vi "SendToSMGR.vi"(6 "error in":errorcluster, 7 "meas_point":i32, 8 "Files":path[](array[path]), 9 "max_value_":string[](array[string]) caption="max_values", 10 "microseconds":string="123456.7" caption="usec", 11 "date":string) -> (0 "error out":errorcluster, 2 "body":string, 3 "headers":string, 5 "time_shift":string="6")   [LabVIEW 2010]
uses:
  <vilib>/httpClient/MultipartData.ctl
  lib/Global 2.vi
  <vilib>/httpClient/LabVIEWHTTPClient.lvlib
panel:
  in  "Tab Control":enum32{"Page 1", "Page 2"}(tab)
  out "Array":T1[](array[typedef]) caption="Данные для формы"
  # "Запрос на добавление данных в базу на сервере\n---------------------------------------------------------------\nЕсли в ответе, в хедерсе есть строка \"HTTP/1.1 200 OK\"\nзначит всё действительно сделано правильно"
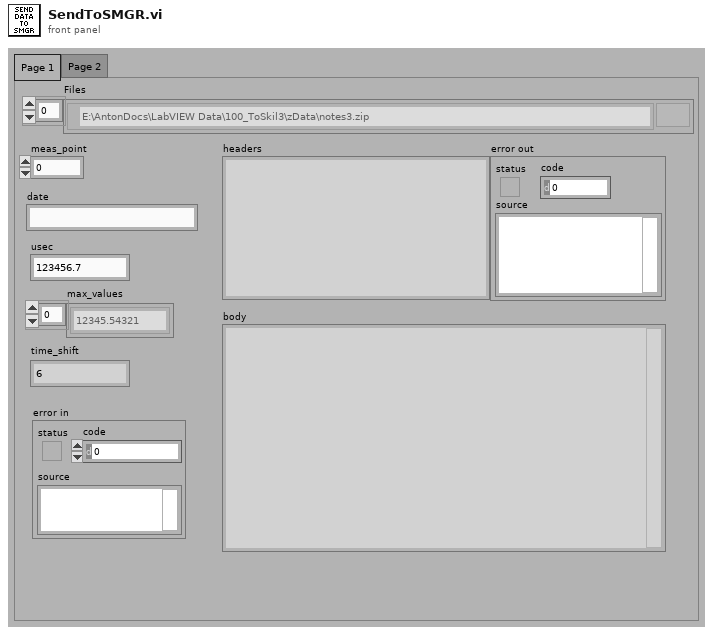
[diagram p1: front panel]
types:
  T1 = typedef "LabVIEWHTTPClient.lvlib/MultipartData.ctl" = cluster{"Name":string, "Value":string, "File":path, "Filename":string, "MIME type":string}
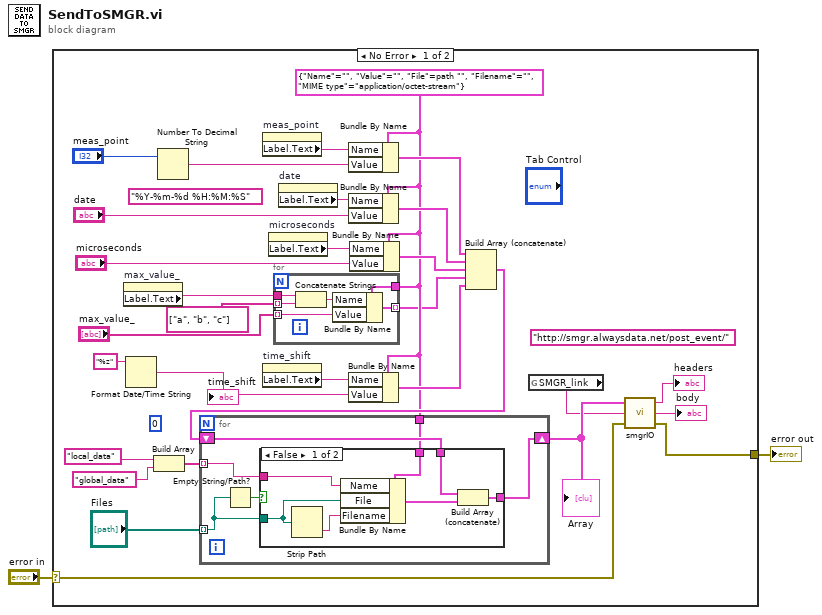
[diagram p0: block diagram]
diagram:
  n1 = case shown="No Error" "error in" {
    selector: "error in" -> [w6 w53]
    tunnel: [w3 w53] -> w1
    frame No Error {
      (unwired) 0
      w12 = T1 {"Name"="", "Value"="", "File"=path "", "Filename"="", "MIME type"="application/octet-stream"} ("postData")
      (unwired) "%Y-%m-%d %H:%M:%S" ("time format string (%c)")
      (unwired) "http://smgr.alwaysdata.net/post_event/" ("URL")
      n2 = property on="max_value_" class="Arr (strict)"() -> ("Label.Text"=w10:string)  [unwired: 2 in, 2 out]
      n3 = Format Date/Time String(time format string (%c)="%z") -> (date/time string=w14:string)  [unwired: 2 in]
      "time_shift" <- w14
      n4 = Build Array("local_data" ("Name"), "global_data" ("Name")) -> (w21:string[])
      n5 = Number To Decimal String(number="meas_point") -> (decimal integer string=w28:string)  [unwired: 1 in]
      n6 = property on="meas_point" class="DigNum (strict)"() -> ("Label.Text"=w19:string)  [unwired: 2 in, 2 out]
      n7 = property on="time_shift" class="Str"() -> ("Label.Text"=w20:string)  [unwired: 2 in, 2 out]
      n8 = property on="microseconds" class="Str"() -> ("Label.Text"=w17:string)  [unwired: 2 in, 2 out]
      n9 = for {
        tunnel: "max_value_" -> [w36] mode=indexing
        tunnel: w12 -> [w38]
        tunnel: [w37] -> w11 mode=indexing
        tunnel: w10 -> [w35]
        tunnel: string[] ["a", "b", "c"] -> [w34] mode=indexing
        n10 = Concatenate Strings(w35, w34) -> (w33:string)
        n11 = Bundle By Name(cluster=w38, "Name"=w33, "Value"=w36) -> (w37:T1)
      }
      n12 = property on="date" class="Str"() -> ("Label.Text"=w18:string)  [unwired: 2 in, 2 out]
      n13 = Bundle By Name(cluster=w12, "Name"=w19, "Value"=w28) -> (w32:T1)
      n14 = Bundle By Name(cluster=w12, "Name"=w18, "Value"="date") -> (w31:T1)
      n15 = Bundle By Name(cluster=w12, "Name"=w20, "Value"=w14) -> (w25:T1)
      n16 = Bundle By Name(cluster=w12, "Name"=w17, "Value"="microseconds") -> (w29:T1)
      n17 = Build Array (concatenate)(w32, w31, w29, w11, w25) -> (w16:T1[])
      n18 = for {
        tunnel: w12 -> [w43]
        tunnel: "Files" -> [w40] mode=indexing
        shift-right: [w42] -> w8
        shift-left: w16 -> [w44]
        tunnel: w21 -> [w41] mode=indexing
        n19 = Empty String/Path?(string/path=w40) -> (empty?=w39:bool)
        n20 = case shown="False" w39 {
          tunnel: w40 -> [w51 _]
          tunnel: w43 -> [w49 _]
          tunnel: w44 -> [w48 w52]
          tunnel: [w46 w52] -> w42
          tunnel: w41 -> [w45 _]
          frame False {
            n21 = Strip Path(path=w51) -> (name=w50:string)  [unwired: 1 out]
            n22 = Bundle By Name(cluster=w49, "Name"=w45, "File"=w51, "Filename"=w50) -> (w47:T1)
            n23 = Build Array (concatenate)(w48, w47) -> (w46:T1[])
          }
          frame True {
          }
        }
      }
      "Array" <- w8
      n24 = global read "Global 2.vi" "SMGR_link"() -> (w7:string)
      n25 = call "smgrIO.vi"("error IO 2"=w6, "URL"=w7, "Array"=w8) -> ("error IO"=w3:errorcluster, "body"=→"body":string, "headers"=→"headers":string)
    }
    frame Error {
    }
  }
  "error out" <- w1
